vi "Count File Levels.vi"(0 "# of Levels In":i32, 1 "String Path":string, 2 "error in (no error)":errorcluster) -> (6 "# of Levels Out":i32, 7 "error out":errorcluster)   [LabVIEW 2017]
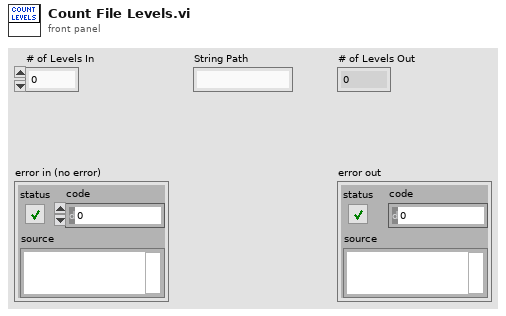
[diagram p1: front panel]
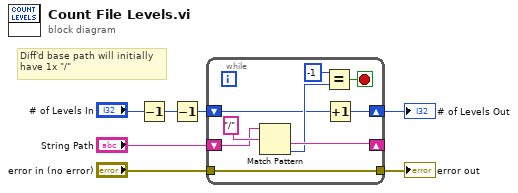
[diagram p0: block diagram]
diagram:
  # "Diff'd base path will initially\nhave 1x \"/\""
  n1 = Decrement(x="# of Levels In") -> (x-1=w2:i32)
  n2 = Decrement(x=w2) -> (x-1=w1:i32)
  n3 = while {
    shift-right: [w14] -> _
    shift-left: "String Path" -> [w15]
    tunnel: "error in (no error)" -> [w12]
    tunnel: [w12] -> w4
    shift-right: [w9] -> w6
    shift-left: w1 -> [w8]
    stop <- w13 stop-if-true
    n4 = Match Pattern(string=w15, regular expression="/" ("search string")) -> (after substring=w14:string, offset past match=w11:i32)  [unwired: 1 in, 2 out]
    n5 = Equal?(x=-1, y=w11) -> (x = y?=w13:bool)
    n6 = Increment(x=w8) -> (x+1=w9:i32)
  }
  "# of Levels Out" <- w6
  "error out" <- w4
